vi "cmc_acquisition_3.vi"() -> ()   [LabVIEW 2010]
doc: "I. Description:\nThis example demonstrates how to continuously acquire data (waveform) using software timing (rate is governed by while loop iteration interval).\n\nII. Instructions for Running:\n1. Select the physical channel to correspond to where your signal is input on the DAQ device.\n2. Enter the minimum and maximum voltage ranges.\nNote: For better accuracy try to match the input range to the expected voltage level of the measured signal.\n\nIII. Block Diagram Steps:\n1. Create an analog input voltage channel.\n2. Call the Start VI to start the task.\n3. Read the waveform data in a loop until the user hits the stop\nbutton or an error occurs.\n4. Call the Clear Task VI to clear the Task.\n5. Use the popup dialog box to display an error if any.\n\nIV. I/O Connections Overview:\nMake sure your signal input terminal matches the Physical Channel I/O control."
uses:
  <vilib>/Utility/error.llb/DialogType.ctl
  <vilib>/DAQmx/read.llb/DAQmx Read (Analog DBL 1Chan 1Samp).vi
  <vilib>/DAQmx/create/channels.llb/DAQmx Create Channel (AI-Voltage-Basic).vi
  <vilib>/daqmx/miscellaneous.llb/DAQmx Fill In Error Info.vi
panel:
  in  "units":i32(ring)=10348 items=["Volts"=10348, "SML-10 lbf"=10065]
  in  "Load Limit":dbl min=-10.0 max=10.0
  in  "Scale":tag
  in  "Write to File":bool
  in  "Software Loop Time (ms)":u32=250
  in  "Physical Channel":tag="Dev1/ai0"
  in  "Minimum Value":dbl=-10.0 format="%0.2f"
  in  "Maximum Value":dbl=10.0 format="%0.2f"
  in  "stop":bool
  out "Measurement":dbl(graph)
  # "For instructions, select Help>>Show Context Help"
  # "Timing Parameters"
  # "Channel Parameters"
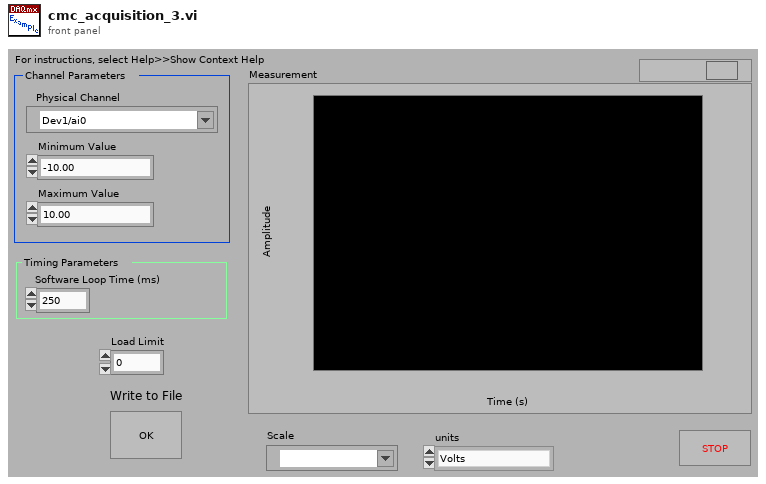
[diagram p1: front panel]
types:
  T1 = enum16{"open", "replace", "create", "open or create", "replace or create", "replace or create with confirmation"}
  T2 = typedef "DialogType.ctl" = u16
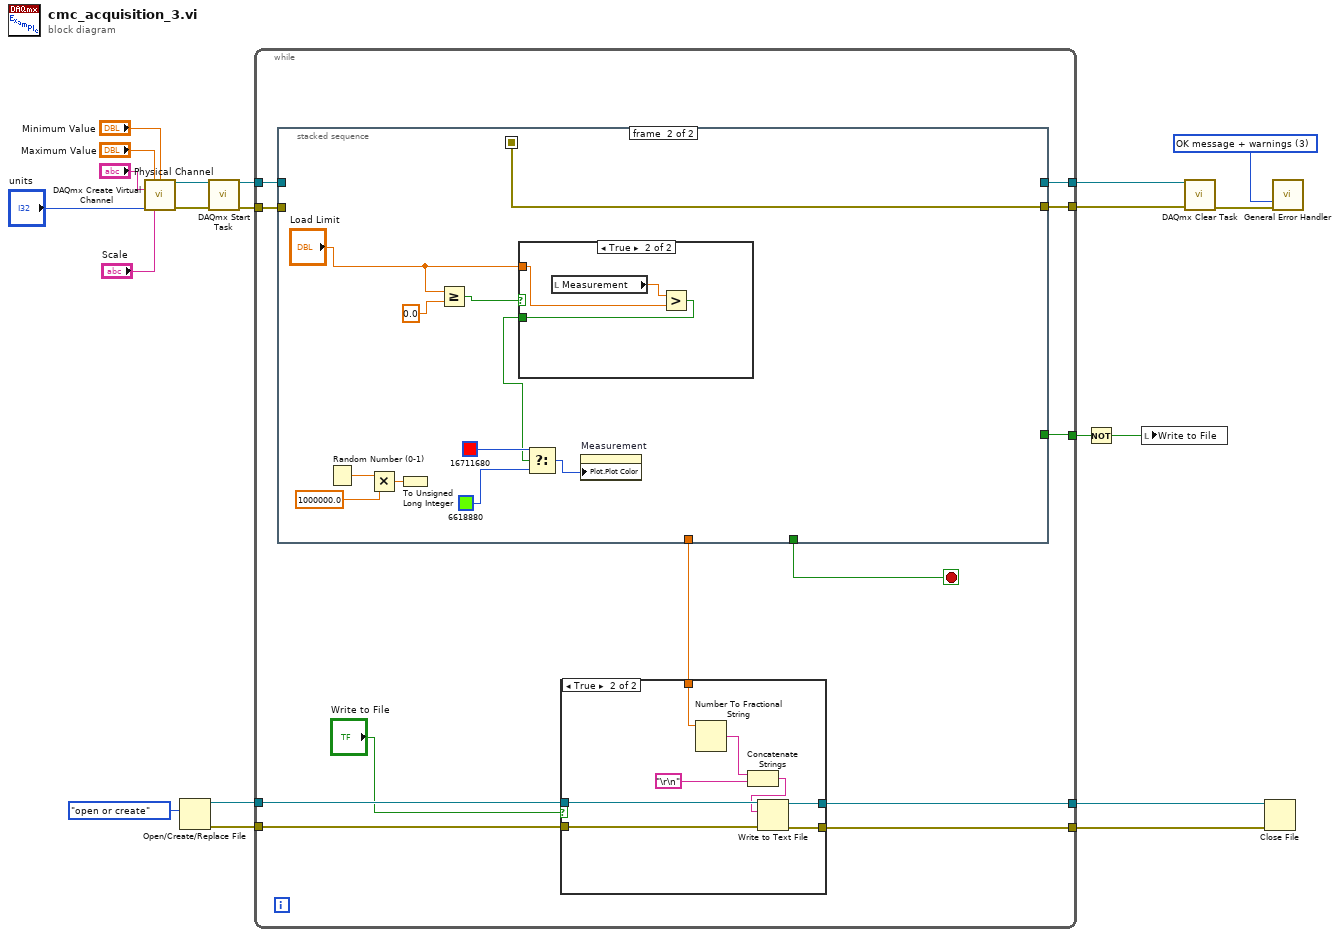
[diagram p0: block diagram]
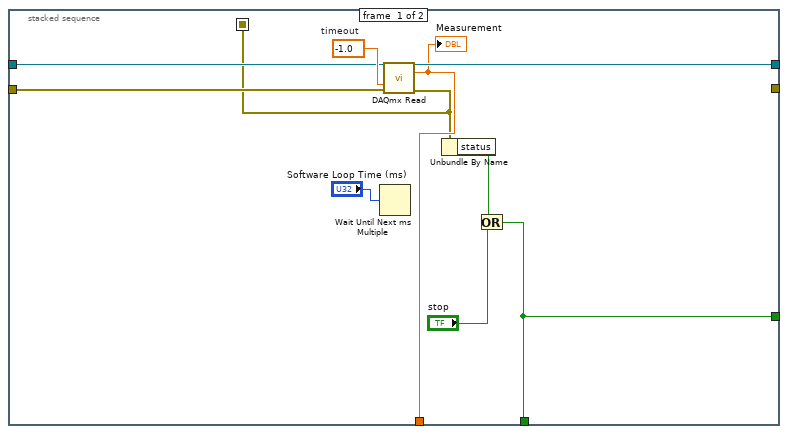
[diagram p2: hidden frame]
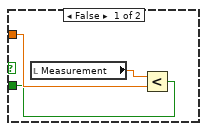
[diagram p3: hidden frame]
diagram:
  w12 = T2 3 items=["no dialog", "OK message", "continue or stop message", "OK message + warnings", "continue/stop + warnings"] ("type of dialog (OK msg:1)")
  n1 = call-poly <vilib>:"DAQmx Create Virtual Channel.vi"("maximum value"="Maximum Value", "minimum value"="Minimum Value", "physical channels"="Physical Channel", "units"="units", "custom scale name"="Scale") -> ("task out"=w14:refnum<k21>, "error out"=w13:errorcluster)  [unwired: 9 in]
  n2 = Open/Create/Replace File(operation (0:open)=T1."open or create") -> (refnum out=w10:refnum<file>, error out=w9:errorcluster)  [unwired: 5 in, 1 out]
  n3 = call <vilib>:"DAQmx Start Task.vi"("task/channels in"=w14, "error in"=w13) -> ("task out"=w17:refnum<k21>, "error out"=w4:errorcluster)  [unwired: 12 in]
  n4 = while {
    tunnel: w17 -> [w25]
    tunnel: [w32] -> w16
    tunnel: w10 -> [w31]
    tunnel: w9 -> [w30]
    tunnel: [w29] -> w8
    tunnel: [w28] -> w7
    tunnel: w4 -> [w24]
    tunnel: [w23] -> w3
    tunnel: [w21] -> w2
    stop <- w22 stop-if-true
    n5 = stacked-sequence {
      seq-local: [w34 _] -> [_ w48]
      tunnel: [w40 _] -> w32
      tunnel: [w38 _] -> w27
      tunnel: w25 -> [w36 _]
      tunnel: w24 -> [w35 _]
      tunnel: [_ w48] -> w23
      tunnel: [w33 _] -> w22
      tunnel: [w33 _] -> w21
      frame #0 {
        w37 = -1.0  # timeout
        n6 = Wait Until Next ms Multiple(millisecond multiple="Software Loop Time (ms)") -> ()  [unwired: 1 out]
        n7 = call-poly <vilib>:"DAQmx Read.vi"("task/channels in"=w36, "timeout"=w37, "error in"=w35) -> ("task out"=w40:refnum<k21>, "data"=w38:dbl, "error out"=w34:errorcluster)  [unwired: 10 in]
        "Measurement" <- w38
        n8 = Unbundle By Name(w34) -> ("status"=w41:bool)
        n9 = Or(x=w41, y="stop") -> (x .or. y?=w33:bool)
      }
      frame #1 {
        n10 = Random Number (0-1)() -> (number: 0 to 1=w52:dbl)
        n11 = Multiply(x=w52, y=1000000.0) -> (x*y=w50:dbl)
        n12 = To Unsigned Long Integer(number=w50) -> ()  [unwired: 1 out]
        n13 = Greater Or Equal?(x="Load Limit", y=0.0) -> (x >= y?=w47:bool)
        n14 = case shown="True" w47 {
          tunnel: [w55 w58] -> w44
          tunnel: "Load Limit" -> [w56 w57]
          frame False {
            n15 = local read "Measurement"() -> (w54:dbl)
            n16 = Less?(x=w54, y=w56) -> (x < y?=w55:bool)
          }
          frame True {
            n17 = local read "Measurement"() -> (w59:dbl)
            n18 = Greater?(x=w59, y=w57) -> (0:w58:bool)
          }
        }
        n19 = Select(t=u32 16711680, s=w44, f=u32 6618880) -> (s? t:f=w49:u32)
        n20 = property on="Measurement" class="WFChart (strict)"("Plot.Plot Color"=w49) -> ()  [unwired: 2 in, 2 out]
      }
    }
    n21 = case shown="True" "Write to File" {
      tunnel: w31 -> [w61 w69]
      tunnel: w30 -> [w60 w68]
      tunnel: [w61 w67] -> w29
      tunnel: [w60 w66] -> w28
      tunnel: w27 -> [_ w65]
      frame False {
      }
      frame True {
        n22 = Number To Fractional String(number=w65) -> (F-format string=w64:string)  [unwired: 3 in]
        n23 = Concatenate Strings(w64, "\r\n") -> (w63:string)
        n24 = Write to Text File(file (use dialog)=w69, text=w63, error in=w68) -> (refnum out=w67:refnum<file>, error out=w66:errorcluster)  [unwired: 1 in, 1 out]
      }
    }
  }
  n25 = Not(x=w2) -> (.not. x?=w1:bool)
  n26 = local write "Write to File"(w1) -> ()
  n27 = call <vilib>:"DAQmx Clear Task.vi"("task in"=w16, "error in"=w3) -> ("error out"=w18:errorcluster)  [unwired: 13 in]
  n28 = Close File(refnum=w8, error in=w7) -> ()  [unwired: 2 out]
  n29 = call <vilib>:"General Error Handler.vi"("type of dialog (OK msg:1)"=w12, "error in (no error)"=w18) -> ()  [unwired: 9 in, 5 out]
